vi "Read Actor Events.vi"(11 "Template in":refnum<class "Template.lvclass">) -> (3 "Base Actor Events":T1)   [LabVIEW 2020, in "Template.lvlib" / "Template.lvclass"]
doc: "Returns the actor events cluster"
uses:
  Template.lvclass
  typedefs/base actor events.ctl
  typedefs/actor configuration.ctl
  typedefs/shared actor configuration.ctl
  typedefs/resource config/device configuration cluster.ctl
  typedefs/resource config/single resource cluster.ctl
  Template.lvclass/Template.ctl
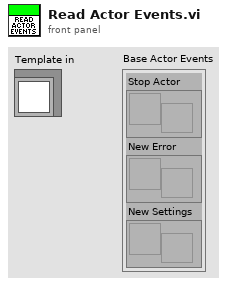
[diagram p1: front panel]
types:
  T1 = typedef "Template.lvlib/Template.lvclass/base actor events.ctl" = cluster{"Stop Actor":refnum<user-event>, "New Error":refnum<user-event>, "New Settings":refnum<user-event>}
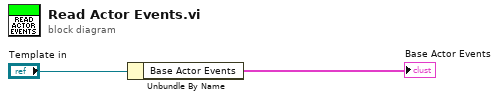
[diagram p0: block diagram]
diagram:
  n1 = Unbundle By Name("Template in") -> ("Base Actor Events"=→"Base Actor Events":T1)
